vi "IsStringAllDigits.vi"(11 "String":string) -> (3 "Boolean":bool)   [LabVIEW 2013, in "BarCodes.lvlib" / "EAN-13.lvclass"]
doc: "Returns whether a VI is composed entirely of digits. This ignores spaces."
uses:
  EAN-13.lvclass
  BarCodes.lvlib
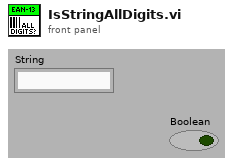
[diagram p1: front panel]
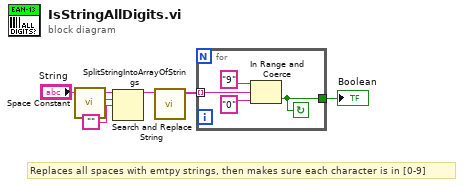
[diagram p0: block diagram]
diagram:
  # "Replaces all spaces with emtpy strings, then makes sure each character is in [0-9]"
  n1 = call <vilib>:"Space Constant.vi"() -> ("String"=w1:string)
  n2 = Search and Replace String(input string="String", search string=w1, replace string="") -> (result string=w3:string)  [unwired: 5 in, 3 out]
  n3 = call "SplitStringIntoArrayOfStrings.vi"("String"=w3) -> ("Characters"=w4:string[])  [unwired: 10 in]
  n4 = for {
    tunnel: w4 -> [w10] mode=indexing
    tunnel: [w7] -> w6
    stop <- w7 continue-if-true
    n5 = In Range and Coerce(upper limit="9" ("lower limit"), x=w10, lower limit="0") -> (In Range?=w7:bool)  [unwired: 1 out]
  }
  "Boolean" <- w6
